vi "Remote Panel Methods Client.vi"() -> ()   [LabVIEW 2015]
doc: "This VI illustrates how to programmatically connect to a remote front panel. A connection is established to the specified VI and control can also be requested. Once control is requested, the VI can only be run once since the server will close the connection automatically after one run."
panel:
  in  "VI Name":string="main_RT.vi"
  in  "Remote Panel Server Port":i32=8000
  in  "Remote Panel Server Address":string="172.22.11.2"
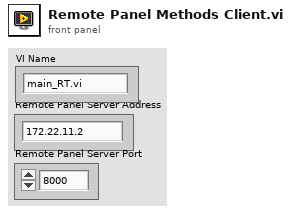
[diagram p1: front panel]
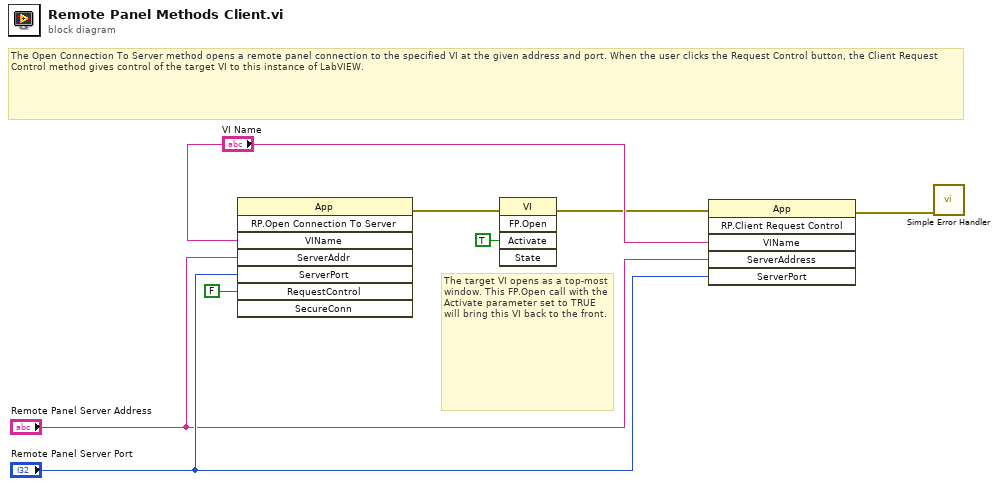
[diagram p0: block diagram]
diagram:
  # "The target VI opens as a top-most window. This FP.Open call with the Activate parameter set to TRUE will bring this VI back to the front."
  # "The Open Connection To Server method opens a remote panel connection to the specified VI at the given address and port. When the user clicks the Request Control button, the Client Request Control method gives control of the target VI to this instance of LabVIEW."
  n1 = invoke class="App" method="RP.Open Connection To Server"("VIName"="VI Name", "ServerAddr"="Remote Panel Server Address", "ServerPort"="Remote Panel Server Port", "RequestControl"=FALSE) -> (error out=w7:errorcluster)  [unwired: 4 in, 7 out]
  n2 = invoke class="VI" method="FP.Open"(error in=w7, "Activate"=TRUE ("Activate?")) -> (error out=w2:errorcluster)  [unwired: 3 in, 4 out]
  n3 = invoke class="App" method="RP.Client Request Control"(error in=w2, "VIName"="VI Name", "ServerAddress"="Remote Panel Server Address", "ServerPort"="Remote Panel Server Port") -> (error out=w6:errorcluster)  [unwired: 2 in, 5 out]
  n4 = call <vilib>:"Simple Error Handler.vi"("error in (no error)"=w6) -> ()  [unwired: 4 in, 5 out]
